vi "Pack for gRPC.vi"(8 "error in":errorcluster, 9 "configuration / results":enum16{"Configuration", "Results"}(ring), 10 "data value":variant, 11 "measurement plugin in":refnum<class "CAN-LIN Raw Bus Capture.lvclass">) -> (0 "error out":errorcluster, 2 "any":T1, 3 "measurement plugin out":refnum<class "CAN-LIN Raw Bus Capture.lvclass">)   [LabVIEW 2025, in "CAN-LIN Raw Bus Capture.lvclass"]
uses:
  CAN-LIN Raw Bus Capture.lvclass
  CAN-LIN Raw Bus Capture.lvclass/CAN-LIN Raw Bus Capture.ctl
  Measurement Configuration.ctl
  Measurement Results.ctl
  a6012965-5700-4384-8228-972e71b6560c.vi
  2eca732d-dbaa-43bf-a7dd-ede2da65bc1b.vi
  <vilib>/Plug-In SDKs/Measurements/Measurement Plugin Service/Measurement Plugin Service.lvclass
  CAN-LIN Raw Bus Capture UI/Toggle.ctl
  <vilib>/gRPC/LabVIEW gRPC Library/Shared/Any.ctl
  <vilib>/gRPC/LabVIEW gRPC Library/grpc-lvsupport-release.lvlib
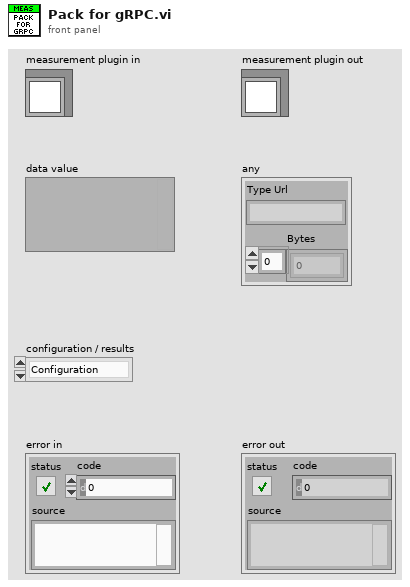
[diagram p1: front panel]
types:
  T1 = typedef "grpc-lvsupport-release.lvlib/Any.ctl" = cluster{"Type Url":string, "Bytes":u8[]}
  T2 = typedef "grpc-lvsupport-release.lvlib/grpcId.ctl" = u64
  T3 = typedef "CAN-LIN Raw Bus Capture.lvclass/Measurement Configuration.ctl" = cluster{"Termination CAN":T4, "FD Baudrate":u32, "Baudrate":u32, "FD ISO Mode":enum32{"ISO", "Legacy ISO", "Non-ISO"}, "IO Mode":enum32{"CAN", "CAN FD", "CAN FD + BRS"}, "Termination LIN":T4, "Can Interface":string, "Lin Interface":string, "Bus Type":string, "INTERFACE NAME CAN":refnum<k21>, "INTERFACE NAME LIN":refnum<k21>, "Timeout (s)":u32}
  T4 = typedef "Toggle.ctl" = bool
  T5 = typedef "CAN-LIN Raw Bus Capture.lvclass/Measurement Results.ctl" = cluster{"Message Buffer":string[][], "Status":string, "OOB gRPC Port":i32, "Connection":bool}
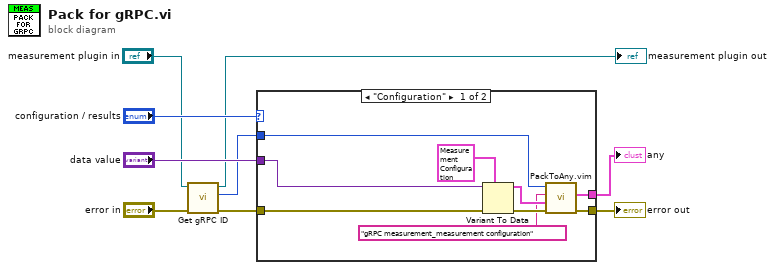
[diagram p0: block diagram]
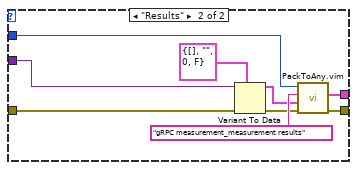
[diagram p2: hidden frame]
diagram:
  n1 = call <vilib>:"Get gRPC ID.vi"("error in"="error in", "measurement plugin service in"="measurement plugin in") -> ("error out"=w4:errorcluster, "gRPC ID"=w1:T2, "measurement plugin service out"=→"measurement plugin out":refnum<class "CAN-LIN Raw Bus Capture.lvclass">)  [unwired: 7 in]
  n2 = case shown="\"Configuration\"" "configuration / results" {
    tunnel: w4 -> [w18 w27]
    tunnel: "data value" -> [w17 w26]
    tunnel: w1 -> [w14 w22]
    tunnel: [w16 w24] -> w8
    tunnel: [w15 w23] -> w7
    frame "Configuration" {
      n3 = Variant To Data(error in=w18, type=T3 {"Termination CAN"=FALSE, "FD Baudrate"=1, "Baudrate"=32, "FD ISO Mode"=enum."Non-ISO", "IO Mode"=enum."CAN FD + BRS", "Termination LIN"=FALSE, "Can Interface"="", "Lin Interface"="", "Bus Type"="", "INTERFACE NAME CAN"="", "INTERFACE NAME LIN"="", "Timeout (s)"=0} ("measurement configuration"), Variant=w17) -> (data=w13:T3, error out=w12:errorcluster)
      n4 = call "PackToAny.vim"("error in"=w12, "Data To Pack"=w13, "Message Type"="gRPC measurement_measurement configuration", "gRPCid in"=w14) -> ("error out"=w16:errorcluster, "Any"=w15:T1)  [unwired: 5 in, 1 out]
    }
    frame "Results" {
      n5 = Variant To Data(error in=w27, type=T5 {"Message Buffer"=[], "Status"="", "OOB gRPC Port"=0, "Connection"=FALSE} ("Measurement Results"), Variant=w26) -> (data=w20:T5, error out=w19:errorcluster)
      n6 = call "PackToAny.vim"("error in"=w19, "Data To Pack"=w20, "Message Type"="gRPC measurement_measurement results", "gRPCid in"=w22) -> ("error out"=w24:errorcluster, "Any"=w23:T1)  [unwired: 5 in, 1 out]
    }
  }
  "error out" <- w8
  "any" <- w7
